vi "Edit Pre Build Help VI Constant.vi"(7 "template base name":string, 8 "error in":errorcluster, 9 "CD name":string, 10 "relative path of VI to edit":path, 11 "custom device path":path) -> (0 "error out":errorcluster, 3 "custom device path out":path)   [LabVIEW 2020, in "Template Tool.lvlib"]
uses:
  Template Tool.lvlib
  <vilib>/Utility/traverseref.llb/TRef TravTarget.ctl
  <vilib>/Utility/traverseref.llb/VI Scripting - Traverse.lvlib
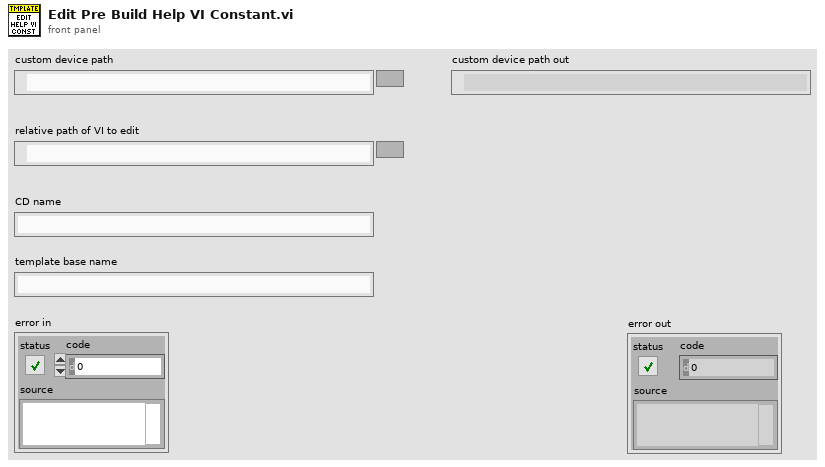
[diagram p1: front panel]
types:
  T1 = typedef "TRef TravTarget.ctl" = enum16{"FP", "BD", "Other"}
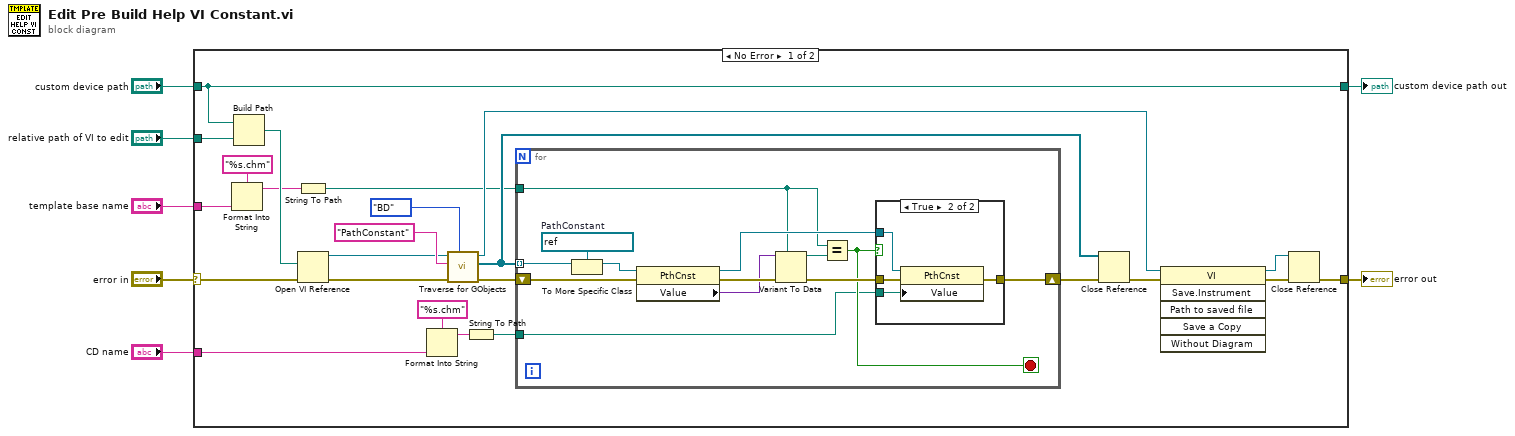
[diagram p0: block diagram]
diagram:
  n1 = case shown="No Error" "error in" {
    selector: "error in" -> [w27 w50]
    tunnel: [w23 w50] -> w7
    tunnel: "custom device path" -> [w28 w51]
    tunnel: "relative path of VI to edit" -> [w29 _]
    tunnel: [w28 w51] -> w4
    tunnel: "CD name" -> [w12 _]
    tunnel: "template base name" -> [w10 _]
    frame No Error {
      n2 = Format Into String(format string="%s.chm", w10) -> (resulting string=w9:string)  [unwired: 2 in, 1 out]
      n3 = Build Path(base path=w28, name or relative path=w29) -> (appended path=w30:path)
      n4 = String To Path(string=w9) -> (path=w8:path)
      n5 = Open VI Reference(vi path=w30, error in (no error)=w27) -> (vi reference=w20:refnum<vi>, error out=w31:errorcluster)  [unwired: 4 in]
      n6 = Format Into String(format string="%s.chm", w12) -> (resulting string=w14:string)  [unwired: 2 in, 1 out]
      n7 = call <vilib>:"Traverse for GObjects.vi"("Traverse Target"=TRef_TravTarget."BD", "error in (no error)"=w31, "Class Name"="PathConstant", "VI Refnum"=w20) -> ("error out"=w18:errorcluster, "References"=w16:refnum<vi>[], "dup VI Refnum"=w19:refnum<vi>)  [unwired: 4 in, 1 out]
      n8 = String To Path(string=w14) -> (path=w13:path)
      n9 = for {
        shift-right: [w36] -> w17
        shift-left: w18 -> [w41]
        tunnel: w16 -> [w44] mode=indexing
        tunnel: w13 -> [w33]
        tunnel: w8 -> [w32]
        stop <- w35 stop-if-true
        w42 = refnum<vi> refnum  # PathConstant
        n10 = To More Specific Class(target class=w42, reference=w44) -> (specific class reference=w43:refnum<vi>)  [unwired: 1 in, 1 out]
        n11 = property class="PthCnst"(reference=w43, error in=w41) -> (reference out=w34:refnum<vi>, error out=w40:errorcluster, "Value"=w39:variant)
        n12 = Variant To Data(error in=w40, type=w32, Variant=w39) -> (data=w38:path, error out=w37:errorcluster)
        n13 = Equal?(x=w32, y=w38) -> (x = y?=w35:bool)
        n14 = case shown="True" w35 {
          tunnel: w37 -> [w45 w49]
          tunnel: [w45 w48] -> w36
          tunnel: w33 -> [_ w47]
          tunnel: w34 -> [_ w46]
          frame False {
          }
          frame True {
            n15 = property class="PthCnst"(reference=w46, error in=w49, "Value"=w47) -> (error out=w48:errorcluster)  [unwired: 1 out]
          }
        }
      }
      n16 = Close Reference(reference=w16, error in (no error)=w17) -> (error out=w26:errorcluster)
      n17 = invoke class="VI" method="Save.Instrument"(reference=w19, error in=w26) -> (reference out=w25:refnum<vi>, error out=w24:errorcluster)  [unwired: 4 in, 4 out]
      n18 = Close Reference(reference=w25, error in (no error)=w24) -> (error out=w23:errorcluster)
    }
    frame Error {
    }
  }
  "error out" <- w7
  "custom device path out" <- w4
